vi "Window Comparison.vi"() -> (0 "Frequency Domain":dbl[][](graph)=[[-56.44474372551401, -56.43619029240049, -56.41057567354017, -56.368035514897066, -56.30879131964156, -56.23314385388433, -56.141464420163445, -56.03418444668477, -55.91178389529689, -55.77477900539368, -55.6237098675911, -55.45912826686764, -55.281586158849755, -55.09162505480851, -54.88976649971282, -54.67650374078542, -54.452294606887286, -54.21755555491696, -53.97265678946232, -53.71791832586374, -53.45360684319533, -53.17993316024045, -52.897050161867256, -52.60505100283404, -52.303967418589124, -51.99376797591707, -51.674356098480274, -51.345567701729976, -51.00716826667277, -50.6588491710409, -50.300223077806905, -49.930818152528616, -49.550070840004345, -49.157316873595775, -48.75178011217631, -48.332558692855415, -47.89860784233153, -47.44871849111166, -46.9814905612456, -46.49529941766208, -45.988253437098365, -45.45813988238372, -44.9023551569401, -44.31781386820727, -43.70082864368179, -43.04694880612665, -42.35073993702655, -41.60547645116801, -40.80270262332738, -39.93158834517799, -38.977952647086354, -37.9227257244304, -36.73941132788347, -35.389652006488255, -33.81489131966394, -31.91911246544791, -29.527986009158823, -26.27059688982638, -21.09222634925326, -6.906979943599807, -16.64288464998015, -23.912733569403308, -27.775015982984037, -30.41105599428544, -32.40880505132885, -34.01422091975582, -35.353871403715274, -36.50153122352522, -37.503967603423916, -38.392661534216394, -39.18973898466388, -39.91113583696903, -40.56795801357037, -41.16322335186558, -42.00951596100797, -42.29172287395494, -42.77004807012277, -43.2240770385082, -43.65260237889531, -44.0575027651805, -44.44087572194774, -44.80466319045622, -45.15059647026764, -45.480205180770156, -45.794839831091096, -46.09569544453051, -46.38383294004535, -46.66019761076787, -46.92563483124129, -47.18090334011886, -47.426686470614996, -47.66360166638087, -47.892208571119596, -48.113015931915974, -48.32648751384695, -48.53304718794668, -48.7330833254793, -48.92695260776996, -49.11498334164324, -49.29747835496882, -49.47471753417496, -49.64696005529653, -49.814446351727284, -49.97739985495962, -50.136028538911255, -50.290526293751235, -50.44107415125985, -50.58784138050651, -50.730986469915365, -50.87065800953348, -51.00699548539292, -51.14012999622955, -51.27018490147062, -51.397276408229416, -51.521514104036214, -51.643001441202124, -51.76183617797797, -51.87811078102513, -51.99191279318963, -52.103325170099225, -52.21242658868189, -52.319291730360966, -52.42399154137612, -52.52659347239565, -52.62716169935912, -52.725757327281826, -52.822438578564885, -52.91726096719566, -53.0102774600838, -53.10153862664982, -53.19109277767247, -53.27898609430025, -53.36526274805011, -53.44996501253257, -53.53313336757214, -53.61480659633435, -53.69502187601461, -53.7738148625829, -53.85121977004975, -53.927269444670316, -54.00199543446008, -54.0754280543759, -54.14759644748281, -54.21852864238923, -54.288251607223344, -54.35679130039884, -54.4241727183866, -54.490419940704115, -54.55555617231667, -54.619603783618096, -54.68258434815708, -54.74451867826072, -54.80542685868862, -54.86532827844681, -54.924241660882174, -54.98218509216273, -55.03917604824736, -55.09523142043963, -55.150367539610414, -55.20460019917387, -55.25794467688864, -55.31041575555697, -55.3620277426874, -55.41279448917847, -55.4627294070834, -55.51184548651016, -55.56015531170026, -55.607671076337645, -55.65440459813219, -55.70036733271123, -55.74557038686251, -55.79002453116567, -55.83374021203832, -55.87672756323232, -55.918996416813236, -55.960556313641085, -56.00141651338457, -56.041586004094555, -56.08107351135247, -56.119887507020564, -56.15803621761415, -56.19552763231109, -56.23236951061925, -56.26856938971873, -56.30413459149311, -56.33907222926592, -56.37338921425619, -56.40709226176582, -56.440187897112956, -56.47268246132049, -56.504582116573644, -56.535892851456886, -56.56662048597753, -56.59677067638852, -56.626348919820124, -56.65536055872436, -56.68381078514413, -56.71170464481645, -56.73904704111138, -56.76584273881515, -56.79209636777191, -56.817812426377, -56.84299528493676, -56.86764918890067, -56.8917782619646, -56.915386509055836, -56.93847781920481, -56.961055968303214, -56.983124621757284, -57.004687337040075, -57.02574756614362, -57.04630865793726, -57.06637386043602, -57.08594632297977, -57.105029098329055, -57.123625144679494, -57.14173732759674, -57.159368421877474, -57.176521113335674, -57.19319800051856, -57.20940159635575, -57.225134329740754, -57.240398547048386, -57.25519651359341, -57.26953041502533, -57.28340235866723, -57.29681437479993, -57.30976841788831, -57.32226636775593, -57.33431003071068, -57.3459011406166, -57.357041359918014, -57.36773228061952, -57.377975425215205, -57.387772247574745, -57.39712413378776, -57.406032402961586, -57.414498307978626, -57.422523036214635, -57.430107710213704, -57.43725338832558, -57.44396106530506, -57.450231672871794, -57.45606608023428, -57.461465094576994, -57.466429461510586, -57.470959865488766, -57.47505693018755, -57.478721218851526, -57.48195323460655, -57.48475342073695, -57.48712216092975, -57.48905977948796, -57.49056654150701, -57.491642653021, -57.49228826111739], [-128.6464243614435, -128.61964439161093, -128.5397395221037, -128.40797875077325, -128.22636259813723, -127.99747061948337, -127.72428121701181, -127.40998681333164, -127.0578237411936, -126.67092995346786, -126.25223672855243, -125.80439471733592, -125.32973072622022, -124.83022946109281, -124.30753381856385, -123.76295777684436, -123.19750685870082, -122.61190222587092, -122.00660556761811, -121.38184286119471, -120.73762575816163, -120.07376988402514, -119.38990971018741, -118.6855098569358, -117.95987280551014, -117.21214307117462, -116.44130788411218, -115.64619436112383, -114.82546310950043, -113.97759811881744, -113.1008926504454, -112.19343070477674, -111.2530634939476, -110.27738009191498, -109.26367115898285, -108.20888430599821, -107.10956915644871, -105.9618095198895, -104.76113925109546, -103.50243714709231, -102.17979452282646, -100.78634671344912, -99.31405620917997, -97.75342986041188, -96.09314464033126, -94.31954405078696, -92.415947414779, -90.361681645281, -88.13068933484607, -85.6894679071259, -82.99390987358979, -79.9842498303537, -76.57655327444758, -72.6474056938685, -68.00387798262747, -62.31707442262347, -54.94574552880933, -44.28994425369213, -21.838162511347903, -12.377837789275281, -15.36392242587983, -36.39575461711411, -50.32597018254913, -58.98236032319505, -65.38017396036554, -70.47987450923733, -74.72767337744185, -78.37039250558895, -81.55920231812743, -84.39181942205585, -86.92818179327435, -89.17136092711196, -90.73923586172054, -77.69591885471812, -71.75447231175538, -79.72381348218407, -99.50652303265363, -100.41133161729687, -101.67096842280385, -102.9598109375992, -104.21586860810194, -105.42548054920391, -106.58676714856183, -107.7013050210499, -108.77171264036043, -109.8008377211495, -110.79146243253616, -111.74619748890466, -112.66745072834073, -113.5574261742604, -114.41813537358394, -115.25141314505048, -116.05893424102317, -116.84222937149235, -117.60269998995646, -118.34163164986902, -119.06020591927125, -119.75951095473718, -120.44055087063286, -121.10425402359323, -121.75148033745816, -122.383027798694, -122.99963822400497, -123.60200237571243, -124.19076452074584, -124.76652650982186, -125.32985141539983, -125.88126678472187, -126.42126758191645, -126.95031882563852, -127.46885795112928, -127.97729697203307, -128.4760244295333, -128.96540713577787, -129.4457917897425, -129.91750644368898, -130.38086180989788, -130.8361524864588, -131.2836580784832, -131.72364419390738, -132.15636338246415, -132.58205600881274, -133.00095101946698, -133.4132666736749, -133.81921122734485, -134.21898353653526, -134.61277363041276, -135.00076325162186, -135.38312633845717, -135.76002948131773, -136.131632346816, -136.49808807482452, -136.85954364200745, -137.21614019733303, -137.56801339049224, -137.91529367138241, -138.25810654758448, -138.5965728651086, -138.9308090543002, -139.26092733109346, -139.58703593085838, -139.90923932479313, -140.22763836275087, -140.54233048369844, -140.85340989166082, -141.16096767267354, -141.46509196561846, -141.76586812056132, -142.0633787866487, -142.3577040555587, -142.64892159872227, -142.9371067407155, -143.22233257350194, -143.5046700802622, -143.78418818805363, -144.06095387331706, -144.33503225634954, -144.60648665396866, -144.87537866462563, -145.14176824444914, -145.4057137551282, -145.66727204253016, -145.92649847756354, -146.18344701921137, -146.4381702754123, -146.69071952256385, -146.9411447670103, -147.18949480825356, -147.43581722217579, -147.68015843518586, -147.92256377673067, -148.1630774444115, -148.40174256819833, -148.63860127474553, -148.87369461704284, -149.10706264882896, -149.33874447307778, -149.568778160405, -149.79720082361035, -150.0240486429249, -150.24935679444025, -150.47315949823792, -150.69549003342837, -150.91638067037377, -151.13586269960413, -151.3539664258439, -151.57072111042626, -151.7861549709433, -152.0002951498191, -152.21316768868058, -152.4247974627841, -152.63520816084545, -152.8444222205125, -153.05246079657326, -153.2593436493876, -153.46508911013254, -153.66971401755774, -153.87323358796334, -154.0756613003412, -154.27700893445405, -154.47728624836938, -154.67650098563115, -154.87465876680434, -155.07176281140713, -155.26781386692812, -155.46281007179263, -155.6567466536565, -155.84961579609785, -156.04140647038298, -156.23210408203235, -156.4216902935657, -156.61014281069643, -156.79743496704657, -156.98353552015072, -157.1684083372541, -157.35201198746768, -157.5342994621913, -157.7152177826393, -157.89470759008003, -158.07270280418163, -158.2491301766799, -158.4239088695865, -158.59695011815427, -158.76815669126233, -158.93742256845317, -159.1046325671641, -159.26966184702758, -159.43237564784468, -159.5926290491458, -159.7502665290654, -159.90512190939296, -160.0570182903499, -160.20576782746144, -160.35117199744465, -160.49302184154845, -160.63109813553697, -160.76517207374394, -160.89500602447856, -161.0203542317227, -161.14096407057093, -161.25657741439394, -161.3669320169997, -161.47176343414685, -161.57080698169943, -161.66379985819975, -161.75048365088605, -161.83060675290758, -161.90392705750662, -161.97021473235617, -162.02925484630083, -162.0808501216089, -162.1248236168995, -162.16102090751477, -162.18931246239237, -162.20959555558298, -162.22179554263954]])   [LabVIEW 2009]
doc: "This example demonstrates the importance of using windows when performing spectral analysis on signals which contain multiple frequencies."
uses:
  <vilib>/Analysis/2dsp.llb/Power Spectrum (DBL).vi
  <vilib>/Analysis/4window.llb/Hanning Window (DBL).vi
  <vilib>/Analysis/4window.llb/Hamming Window (DBL).vi
  <vilib>/Analysis/4window.llb/Triangle Window (DBL).vi
  <vilib>/Analysis/4window.llb/Exact Blackman Window (DBL).vi
  <vilib>/Analysis/4window.llb/Blackman-Harris Window (DBL).vi
  <vilib>/Analysis/4window.llb/Kaiser-Bessel Window (DBL).vi
  <vilib>/Analysis/NI_AALBase.lvlib
  <vilib>/Analysis/NI_AALPro.lvlib
panel:
  in  "window 2":T1(ring)=enum."Hanning"
  in  "window 1":T1(ring)
  in  "Frequency 2":dbl(knob)=59.24467057315707 scale=0.0..100.0 scale format="%.1f"
  in  "Amplitude 2":dbl=1.0 format="%.3f"
  in  "Amplitude 1":dbl=0.0009999999999998899 format="%.3f"
  in  "Frequency 1":dbl(knob)=73.91896097250746 scale=0.0..100.0 scale format="%.1f"
  in  "?":bool
  out "Time Domain":dbl[](graph)=[0.0, 0.6654498491683241, 0.9941672384384495, 0.8198679555361532, 0.2308447441457715, -0.47479668228860833, -0.940069632384146, -0.9297428672376677, -0.44925159343998383, 0.25821463922358356, 0.8348489231284805, 0.9891994150471626, 0.6434379211727421, -0.027457081268967985, -0.6842834348286945, -0.9950944160758938, -0.8029005979646191, -0.20491429811087655, 0.49662537892816666, 0.9471681505909625, 0.9189787799313205, 0.4262213289261399, -0.28213340128497827, -0.8480444969421104, -0.9853263362469421, -0.6243742646453413, 0.052497577796575566, 0.703082960142592, 0.9982676742324846, 0.7885474890916643, 0.17980763783273104, -0.5200919332898787, -0.9570149645685516, -0.9097847432607273, -0.40220440284331055, 0.30891782290151315, 0.8637308337220347, 0.9814968524445173, 0.602688459503532, -0.08092938180146424, -0.7234284840220865, -0.9998221835915982, -0.7704665975917224, -0.15157905953548262, 0.543710609455989, 0.9638295716020571, 0.8965232037716288, 0.3760377153940697, -0.33435874987920433, -0.8755542259707675, -0.9740895570674739, -0.580273447235011, 0.10679495486487493, 0.7398680636822015, 0.9989949989097774, 0.7531696441332307, 0.12655323578821395, -0.5641959815975648, -0.9698846422680215, -0.8852781823951236, -0.3529464539376336, 0.3580979831854206, 0.8882937894157351, 0.9693481832024873, 0.5600436318437855, -0.13274334411112176, -0.7585748063145495, -1.0007391037608382, -0.7365856329754038, -0.09969296721432142, 0.587678060768714, 0.9776911544856296, 0.8730119947451779, 0.3266793991811585, -0.38479485183427853, -0.9014340260905225, -0.9619759276708426, -0.5359898684554747, 0.16087706745118494, 0.7761249438924825, 0.9987304667041069, 0.7163469506126988, 0.07194460627566215, -0.6086183043977795, -0.9813676990080236, -0.858015962883473, -0.301015214649478, 0.40808052147552193, 0.9109023345072254, 0.953321809817795, 0.5138481026683641, -0.18547407937251412, -0.7911997153053777, -0.997063154639603, -0.6988165269578243, -0.04705686378977266, 0.6287561087335684, 0.9868019471688002, 0.8458034687175716, 0.2768613992829304, -0.4323455362346191, -0.9230108836474947, -0.9467699465344929, -0.4914769414034349, 0.21255248195604134, 0.8090672632476903, 0.9962064581736578, 0.6793046872066778, 0.018786176218604053, -0.6510890431981309, -0.9914394856274035, -0.8302289464984455, -0.2492034720572585, 0.45761751250322613, 0.9327746570292058, 0.9361490270043318, 0.46625972612695754, -0.2391604220374431, -0.8234692307446092, -0.9913987295031047, -0.6582037142458792, 0.007618860297994742, 0.6695379364257462, 0.9930353230729912, 0.8146049213896206, 0.22437030090618282, -0.479406767556503, -0.9409865946285191, -0.9269237827141719, -0.44413792912893174, 0.263438143774018, 0.8380509175289786, 0.9889879402347416, 0.6396897590828592, -0.033357336431292156, -0.6897512299641648, -0.9973456466890747, -0.8003741355653826, -0.19838605711252008, 0.5040495035511904, 0.9514728225449471, 0.9174701637826876, 0.4192863670673732, -0.2909339268031248, -0.8538179261146994, -0.9846619495548855, -0.617445218799786, 0.06189676763680295, 0.709678381162434, 0.9983729249608347, 0.7821975080982164, 0.17067332677230088, -0.5269131183927981, -0.9579440439103226, -0.9046705407175516, -0.3941552684827774, 0.31550685091731306, 0.8656498546693304, 0.9782505045244063, 0.5963815603602961, -0.08701191373299944, -0.7265561503915586, -0.9989344103091662, -0.7663088725407743, -0.14609820422929257, 0.5482313291627952, 0.9655499919326439, 0.894634327676418, 0.37112395517330454, -0.3403303424411082, -0.8798309935048296, -0.9743200499818441, -0.5758414475266431, 0.11407508510753216, 0.7463410400964541, 1.0009928889173634, 0.7491697261162099, 0.118341538075631, -0.5722460584650432, -0.9731934567097893, -0.8817664371943493, -0.34439850980425923, 0.3669429536101744, 0.892458221363742, 0.9665208187010624, 0.5519059801247982, -0.14156064637870133, -0.7632295203639651, -0.998920470974981, -0.7296497878151296, -0.09164195882378523, 0.5925999208418719, 0.9772764123405572, 0.8679901379468, 0.3199487960396116, -0.3899082049626558, -0.9027987914153427, -0.9593841917309908, -0.5308919220140453, 0.1662133818986288, 0.7795228448791199, 0.9988042885530354, 0.7129473928600683, 0.06632022459061068, -0.6140910697494728, -0.9840270025681007, -0.856179432069962, -0.2950899591908715, 0.41540318184534186, 0.9157735548123601, 0.9527935109458044, 0.5077360426658705, -0.1941504636969456, -0.7976893602017731, -0.9975650522287463, -0.6928006063644147, -0.03774420989710365, 0.636159480256915, 0.9881191276185818, 0.8403314501904064, 0.26775492767729386, -0.4399669273828236, -0.9250468355110724, -0.9424018961390673, -0.48342000482069913, 0.21981127696106334, 0.8118549380236254, 0.9935231801176485, 0.6730145851359295, 0.012285142431082533, -0.6547557426274477, -0.9909310946935874, -0.8261928745016488, -0.24364814492422932, 0.46231325244007204, 0.9347339087042424, 0.9345637140428507, 0.4616589115992905, -0.24496870339155408, -0.8279140084894399, -0.9921649250018043, -0.6544545891370045, 0.01447353442091208, 0.6761814253483793, 0.9958062339565407, 0.8115805102511681, 0.21673929352703228, -0.48768363911123686, -0.9452576384972791, -0.9245566212040238, -0.43621355829005953, 0.2725828611338932, 0.8432694350810539, 0.9873275426127125, 0.6321256580304697, -0.04251926031574855, -0.6954210674237403, -0.9965741541960247, -0.793907129787096, -0.1900141076893892, 0.5098074525318806, 0.9518737226542175, 0.9128044099044431, 0.4123522288116216, -0.2965823640892201, -0.8557045134487976, -0.9823486083434403, -0.6123572170936948, 0.06738771717657294, 0.7132988937575796, 0.9987109844833099, 0.7790948226256208, 0.1652956494507008, -0.5323557935152977, -0.9609237747367548, -0.9034474511490176, -0.38883635427376506, 0.32262898785000343, 0.8709513370956021, 0.9786258113390705, 0.5911400273657219, -0.095412166153807, -0.733603418528618, -1.0005474632279623, -0.7612981832459339, -0.1370545645588582, 0.5562906439869195, 0.9680593432690078, 0.8901648758301011, 0.36222898587374375, -0.3486316837138593, -0.8829919428914108, -0.9708333510449033, -0.5679314937296321, 0.12193128511308737, 0.750044146005635, 0.9989913596393628, 0.7429978087925168, 0.111442462638001, -0.5765086616102463, -0.9731403472855003, -0.8778861095029407, -0.3387456328644475, 0.3718575218504711, 0.8946700519763989, 0.9652052911829314, 0.5475695747063355, -0.14721453007273969, -0.7677860163935322, -1.0001332108184573, -0.7265324458929228, -0.08525352363862503, 0.5992932746033078, 0.9806982004933998, 0.8659093616589829, 0.3129925991595983, -0.3982452036302915, -0.9079039418564374, -0.9581640081771609, -0.5237295042363151, 0.1754724114032512, 0.7856867611941624, 0.9983519263984749, 0.7061191010615712, 0.05698742273070083, -0.6207049338184426, -0.9843748686285063, -0.8503398171437632, -0.28653185071219817, 0.42197077188334947, 0.917075647070625, 0.9486097755319001, 0.5006757340204673, -0.20034702281332759, -0.8001727369638677, -0.9955994076560585, -0.68773644755774, -0.03206167425481087, 0.640042755983138, 0.9887203725960102, 0.8374831843621632, 0.2625847717219219, -0.44536629687803186, -0.9282751491802019, -0.9417115101799749, -0.47868805800487907, 0.2266582512034026, 0.817457049130033, 0.9947074422333878, 0.6686605909542267, 0.004292171645801479, -0.6621968342032062, -0.9935714497467142, -0.8222474182668593, -0.2350437635186668, 0.4708596490654523, 0.9383815323851941, 0.931194345000516, 0.45315820318107297, -0.253804380044188, -0.8321851818954453, -0.9896778657408049, -0.6468566210336391, 0.022826297515664194, 0.6808215479172248, 0.9946010748389618, 0.8056464376175693, 0.20948783679255928, -0.4925863672825691, -0.9457441440212009, -0.9208872784805545, -0.43045603146439354, 0.27776209609824826, 0.8457652730959259, 0.9862660165181151, 0.6280077825118784, -0.04804335554887082, -0.700054612549675, -0.9981536923062254, -0.7913585357904779, -0.18410723415180635, 0.5164495215928477, 0.9558215849891797, 0.911610721881266, 0.4061356049840273, -0.30482483403373406, -0.861500243819343, -0.9822450278343963, -0.6060683492214182, 0.07657678349830396, 0.7202737450552383, 0.9994732463311157, 0.7731459826440308, 0.15597596261022337, -0.5398113667529439, -0.9624337412141074, -0.8983867762123707, -0.3802461291618335, 0.32994950637570414, 0.873221253857288, 0.9750551692947566, 0.5840543907282498, -0.10214700482885025, -0.7367533684605162, -0.9990137186549296, -0.7562934018071918, -0.13115399025340221, 0.560485507700075, 0.9689426063783679, 0.8875424894099186, 0.3572228645860474, -0.3539941638623834, -0.8864159418992362, -0.9705968266138811, -0.5637487515641929, 0.12845384855414116, 0.7558296238601604, 1.0008781572684484, 0.7395195944738437, 0.1039630288828465, -0.5841815966518887, -0.9767001621913151, -0.8750325953579781, -0.3307321965546422, 0.38071207570407206, 0.8993701134140897, 0.9630024057229065, 0.5396377296697666, -0.15641865387692164, -0.7731189350837357, -0.9987411795887805, -0.7194150681029652, -0.07653119962922568, 0.6048632394404225, 0.9803933867380874, 0.8603465163677918, 0.3054604775936764, -0.4038142148809267, -0.9090171726645675, -0.9547805283616425, -0.5178799087523787, 0.18095828698664418, 0.7885123346372833, 0.997548426308825, 0.7021821014322284, 0.051557695950798, -0.6254022206228804, -0.9862555576006926, -0.8482910214509528, -0.2810990121592954, 0.42848290855987203, 0.9214285861963825, 0.948226955217406, 0.49523368843173593, -0.20835799469092786, -0.8065068845397874, -0.9965520306964414, -0.6824025027611575, -0.02311854056041365, 0.6476738540770295, 0.9906691806193794, 0.8325330301396427, 0.2534653569522363, -0.45353316903736596, -0.9309574004810222, -0.9375674322315831, -0.4702335118718619, 0.23464479944063332, 0.8207372685924307, 0.9918796742968595, 0.6616711727076642, -0.0029453534706681906, -0.6660718343767812, -0.9925641523399849, -0.8173596771661858, -0.228914221949581, 0.47541809094397103, 0.9395839181050798, 0.9287867597137605, 0.4482742082250748, -0.25915250612141705, -0.8357726416882119, -0.9898239674509731, -0.6431721779476549, 0.029000008905983185, 0.6866902149584144, 0.9970787204953082, 0.8030067501544166, 0.2026006943883926, -0.5003376654076918, -0.9500973544556998, -0.9191195719938553, -0.42316134787936116, 0.28674301158736604, 0.8514037098671435, 0.9852623438079504, 0.6208043206587227, -0.05743591262651221, -0.7063679256968324, -0.9979241630394187, -0.7848869175864857, -0.17516471094521563, 0.5229112313922573, 0.9565041207031759, 0.9065605985672192, 0.3984198908460941, -0.3110636623347338, -0.8633239346699696, -0.9792389692684903, -0.600161383356782, 0.08240162385456966, 0.7234845737948822]
  # "Sine Wave 1 + Sine Wave 2"
  # "Sine Wave 1"
  # "Sine Wave 2"
  # "dB"
  # "The effects of different types of window functions is shown in the frequency domain. With no window function used, Sine Wave 2 buries the low amplitude Sine Wave 1.  Using the Hanning Window (Window 2), the smaller signal can be detected."
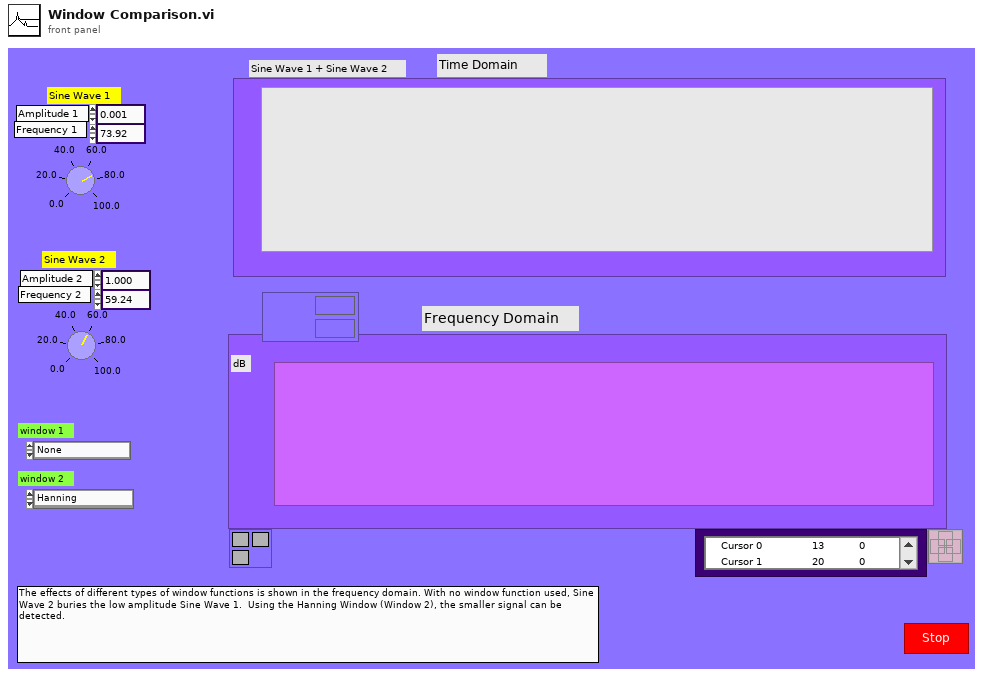
[diagram p1: front panel]
types:
  T1 = enum16{"None", "Hanning", "Hamming", "Triangle", "Exact Blackman", "Blackman-Harris", "Kaiser-Bessel"}
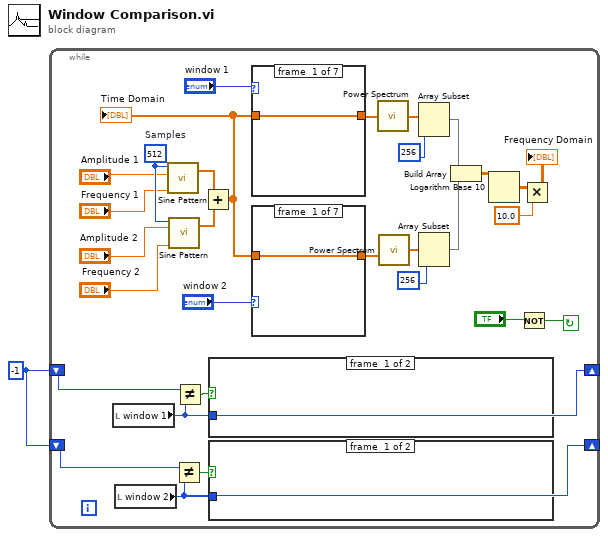
[diagram p0: block diagram]
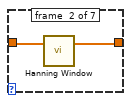
[diagram p2: hidden frame]
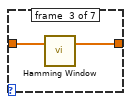
[diagram p3: hidden frame]
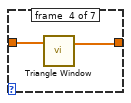
[diagram p4: hidden frame]
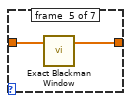
[diagram p5: hidden frame]
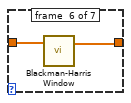
[diagram p6: hidden frame]
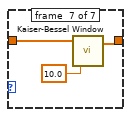
[diagram p7: hidden frame]
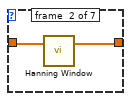
[diagram p8: hidden frame]
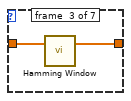
[diagram p9: hidden frame]
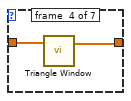
[diagram p10: hidden frame]
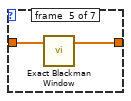
[diagram p11: hidden frame]
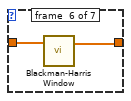
[diagram p12: hidden frame]
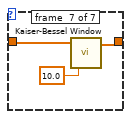
[diagram p13: hidden frame]
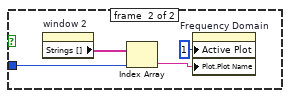
[diagram p14: hidden frame]
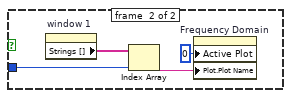
[diagram p15: hidden frame]
diagram:
  w1 = -1
  n1 = while {
    shift-left: w1 -> [w10]
    shift-right: [w8] -> _
    shift-left: w1 -> [w11]
    shift-right: [w9] -> _
    stop <- w27 continue-if-true
    w20 = 512  # Samples
    n2 = local read "window 1"() -> (w9:T1)
    n3 = local read "window 2"() -> (w8:T1)
    n4 = call <vilib>:"Sine Pattern.vi"("cycles"="Frequency 1", "amplitude"="Amplitude 1", "samples"=w20) -> ("Sinusoidal Pattern"=w26:dbl[])  [unwired: 1 in, 1 out]
    n5 = call <vilib>:"Sine Pattern.vi"("cycles"="Frequency 2", "amplitude"="Amplitude 2", "samples"=w20) -> ("Sinusoidal Pattern"=w25:dbl[])  [unwired: 1 in, 1 out]
    n6 = Not Equal?(x=w10, y=w8) -> (x != y?=w23:bool)
    n7 = Not Equal?(x=w11, y=w9) -> (x != y?=w24:bool)
    n8 = Add(x=w26, y=w25) -> (x+y=w4:dbl[])
    "Time Domain" <- w4
    n9 = case shown="True" w24 {
      tunnel: w9 -> [_ w64]
      frame #0 {
      }
      frame #1 {
        n10 = property on="window 1" class="Enum (strict)"() -> ("Strings []"=w66:string[])  [unwired: 2 in, 2 out]
        n11 = Index Array(array=w66, index=w64) -> (element=w65:string)
        n12 = property on="Frequency Domain" class="WaveformGraph (strict)"("Active Plot"=0, "Plot.Plot Name"=w65) -> ()  [unwired: 2 in, 2 out]
      }
    }
    n13 = case shown="True" w23 {
      tunnel: w8 -> [_ w62]
      frame #0 {
      }
      frame #1 {
        n14 = property on="window 2" class="Enum (strict)"() -> ("Strings []"=w61:string[])  [unwired: 2 in, 2 out]
        n15 = Index Array(array=w61, index=w62) -> (element=w60:string)
        n16 = property on="Frequency Domain" class="WaveformGraph (strict)"("Active Plot"=1, "Plot.Plot Name"=w60) -> ()  [unwired: 2 in, 2 out]
      }
    }
    n17 = case shown="\"Kaiser-Bessel\"" "window 1" {
      tunnel: w4 -> [w46 w48 w50 w52 w54 w56 w58]
      tunnel: [w46 w47 w49 w51 w53 w55 w57] -> w3
      frame #0 {
      }
      frame #1 {
        n18 = call-poly <vilib>:"Hanning Window.vi"("X"=w48) -> ("Windowed X"=w47:dbl[])  [unwired: 1 out]
      }
      frame #2 {
        n19 = call-poly <vilib>:"Hamming Window.vi"("X"=w50) -> ("Windowed X"=w49:dbl[])  [unwired: 1 out]
      }
      frame #3 {
        n20 = call-poly <vilib>:"Triangle Window.vi"("X"=w52) -> ("Windowed X"=w51:dbl[])  [unwired: 1 out]
      }
      frame #4 {
        n21 = call-poly <vilib>:"Exact Blackman Window.vi"("X"=w54) -> ("Windowed X"=w53:dbl[])  [unwired: 1 out]
      }
      frame #5 {
        n22 = call-poly <vilib>:"Blackman-Harris Window.vi"("X"=w56) -> ("Windowed X"=w55:dbl[])  [unwired: 1 out]
      }
      frame #6 {
        n23 = call-poly <vilib>:"Kaiser-Bessel Window.vi"("beta"=10.0, "X"=w58) -> ("Windowed X"=w57:dbl[])  [unwired: 1 out]
      }
    }
    n24 = case shown="\"Kaiser-Bessel\"" "window 2" {
      tunnel: w4 -> [w32 w34 w36 w38 w40 w42 w43]
      tunnel: [w32 w33 w35 w37 w39 w41 w45] -> w2
      frame #0 {
      }
      frame #1 {
        n25 = call-poly <vilib>:"Hanning Window.vi"("X"=w34) -> ("Windowed X"=w33:dbl[])  [unwired: 1 out]
      }
      frame #2 {
        n26 = call-poly <vilib>:"Hamming Window.vi"("X"=w36) -> ("Windowed X"=w35:dbl[])  [unwired: 1 out]
      }
      frame #3 {
        n27 = call-poly <vilib>:"Triangle Window.vi"("X"=w38) -> ("Windowed X"=w37:dbl[])  [unwired: 1 out]
      }
      frame #4 {
        n28 = call-poly <vilib>:"Exact Blackman Window.vi"("X"=w40) -> ("Windowed X"=w39:dbl[])  [unwired: 1 out]
      }
      frame #5 {
        n29 = call-poly <vilib>:"Blackman-Harris Window.vi"("X"=w42) -> ("Windowed X"=w41:dbl[])  [unwired: 1 out]
      }
      frame #6 {
        n30 = call-poly <vilib>:"Kaiser-Bessel Window.vi"("beta"=10.0, "X"=w43) -> ("Windowed X"=w45:dbl[])  [unwired: 1 out]
      }
    }
    n31 = call-poly <vilib>:"Power Spectrum.vi"("X"=w3) -> ("Power Spectrum"=w31:dbl[])  [unwired: 1 out]
    n32 = call-poly <vilib>:"Power Spectrum.vi"("X"=w2) -> ("Power Spectrum"=w29:dbl[])  [unwired: 1 out]
    n33 = Array Subset(array=w31, length=256) -> (w18:dbl[])  [unwired: 1 in]
    n34 = Array Subset(array=w29, length=256) -> (w17:dbl[])  [unwired: 1 in]
    n35 = Build Array(w18, w17) -> (w16:dbl[][])
    n36 = Logarithm Base 10(1:w16) -> (0:w21:dbl[][])
    n37 = Not(x="?") -> (.not. x?=w27:bool)
    n38 = Multiply(x=w21, y=10.0) -> (x*y=→"Frequency Domain":dbl[][])
  }
